vi "Desired Color.vi"() -> (1 "Correct Color":bool, 3 "Color to Match":string)   [LabVIEW 2019]
uses:
  Framework/Robot Global Data.vi
  <vilib>/regexp/Match Regular Expression.xnode
panel:
  out "Matched Color Name":string
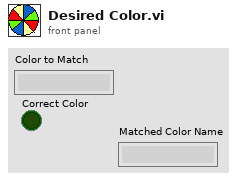
[diagram p1: front panel]
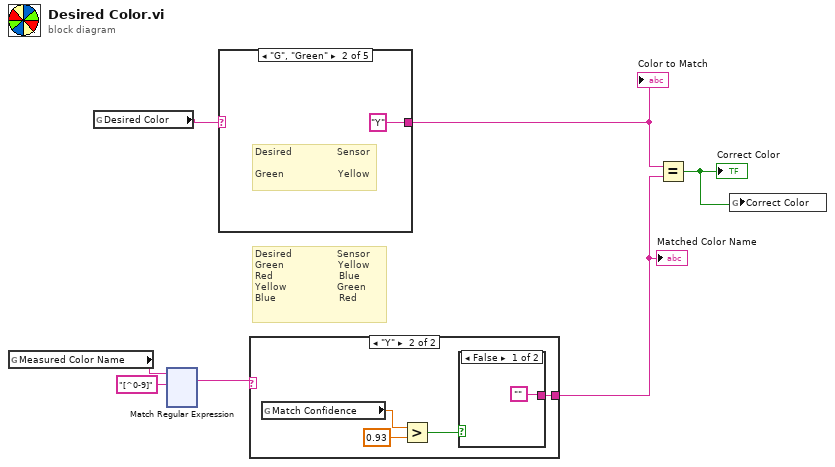
[diagram p0: block diagram]
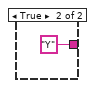
[diagram p3: hidden frame]
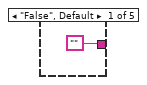
[diagram p4: hidden frame]
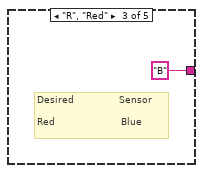
[diagram p5: hidden frame]
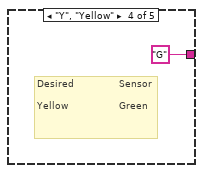
[diagram p6: hidden frame]
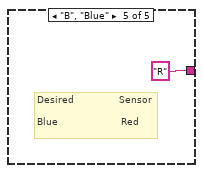
[diagram p7: hidden frame]
diagram:
  # "Desired               Sensor\nGreen                  Yellow\nRed                      Blue       \nYellow                 Green\nBlue                     Red"
  n1 = global read "Robot Global Data.vi" "Measured Color Name"() -> (w5:string)
  n2 = global read "Robot Global Data.vi" "Desired Color"() -> (w7:string)
  n3 = xnode "Match Regular Expression"("input string"=w5, "regular expression"="[^0-9]") -> ("whole match"=w3:string)  [unwired: 4 in, 4 out]
  n4 = case shown="\"G\", \"Green\"" w7 {
    tunnel: ["" "Y" "B" "G" "R"] -> w6
    frame "False", Default {
    }
    frame "G", "Green" {
      # "Desired               Sensor\n\nGreen                  Yellow"
    }
    frame "R", "Red" {
      # "Desired               Sensor\n\nRed                      Blue"
    }
    frame "Y", "Yellow" {
      # "Desired               Sensor\n\nYellow                 Green"
    }
    frame "B", "Blue" {
      # "Desired               Sensor\n\nBlue                     Red"
    }
  }
  "Color to Match" <- w6
  n5 = case shown="\"Y\"" w3 {
    selector: w3 -> [w13 _]
    tunnel: [w13 w14] -> w2
    frame Default {
    }
    frame "Y" {
      n6 = global read "Robot Global Data.vi" "Match Confidence"() -> (w17:dbl)
      n7 = Greater?(x=w17, y=0.93) -> (0:w15:bool)
      n8 = case shown="False" w15 {
        tunnel: ["" "Y"] -> w14
        frame False {
        }
        frame True {
        }
      }
    }
  }
  "Matched Color Name" <- w2
  n9 = Equal?(x=w6, y=w2) -> (x = y?=w1:bool)
  "Correct Color" <- w1
  n10 = global write "Robot Global Data.vi" "Correct Color"(w1) -> ()
